vi "Rename InstrumentStudio Plug-In Main VI.vi"(0 "configuration":T1, 5 "Plugin Library Path":path, 11 "error in":errorcluster) -> (4 "IS Plugin Main VI Path":path, 15 "error out":errorcluster)   [LabVIEW 2021, in "InstrumentStudio Plug-In Editor.lvlib"]
uses:
  InstrumentStudio Plug-In Editor.lvlib
  controls/Data Holder.ctl
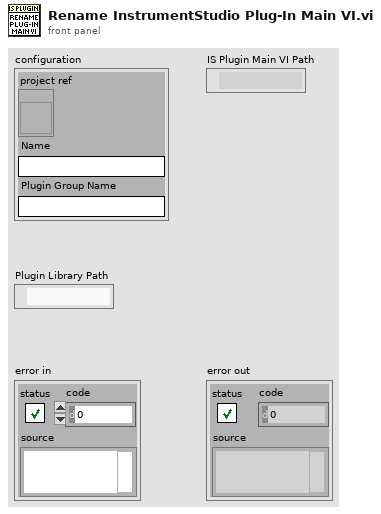
[diagram p1: front panel]
types:
  T1 = typedef "InstrumentStudio Plug-In Editor.lvlib/Data Holder.ctl" = cluster{"project ref":refnum<vi>, "Name":string, "Plugin Group Name":string}
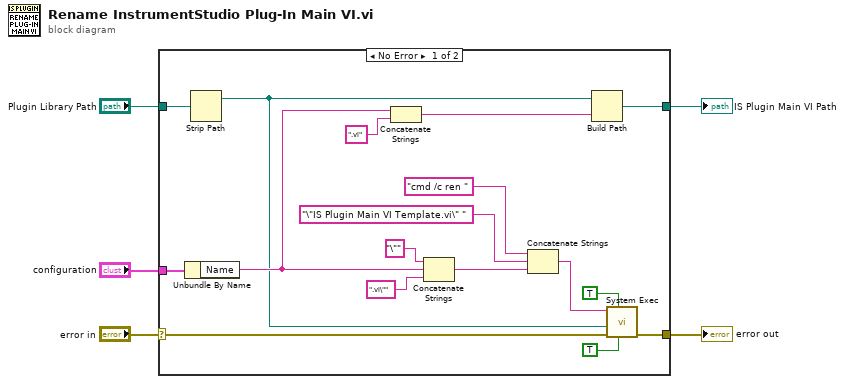
[diagram p0: block diagram]
diagram:
  n1 = case shown="No Error" "error in" {
    selector: "error in" -> [w21 w23]
    tunnel: "configuration" -> [w22 _]
    tunnel: "Plugin Library Path" -> [w10 _]
    tunnel: [w7 _] -> w2
    tunnel: [w6 w23] -> w1
    frame No Error {
      n2 = Unbundle By Name(w22) -> ("Name"=w13:string)
      n3 = Strip Path(path=w10) -> (stripped path=w9:path)  [unwired: 1 out]
      n4 = Concatenate Strings(w13, ".vi" ("string")) -> (w11:string)
      n5 = Concatenate Strings("\"" ("string"), w13, ".vi\"" ("string")) -> (w15:string)
      n6 = Concatenate Strings("cmd /c ren " ("string"), "\"IS Plugin Main VI Template.vi\" " ("string"), w15) -> (w18:string)
      n7 = Build Path(base path=w9, name or relative path=w11) -> (appended path=w7:path)
      n8 = call <vilib>:"System Exec.vi"("run minimized? (F)"=TRUE, "wait until completion? (T)"=TRUE, "error in (no error)"=w21, "working directory"=w9, "command line"=w18) -> ("error out"=w6:errorcluster)  [unwired: 3 in, 3 out]
    }
    frame Error {
    }
  }
  "error out" <- w1
  "IS Plugin Main VI Path" <- w2
